vi "Inst_K2002.vi"(8 "error in":errorcluster, 10 "All Message Queues in":T1, 11 "Prueba31 in":refnum<class "Prueba31.lvclass">) -> (0 "error out":errorcluster)   [LabVIEW 2019, in "Prueba31.lvclass"]
uses:
  Prueba31.lvclass
  QMH/Message Queue/All Message Queues.ctl
  QMH/Message Queue/Message Cluster.ctl
  Prueba31.lvclass/Prueba31.ctl
  <vilib>/Utility/error.llb/Error Cluster From Error Code.vi
  QMH/Message Queue/Enqueue Message (Single).vi
  <vilib>/ErrorRing/Error Ring.xnode
  QMH/Message Queue/Message Queue.lvlib
  Instrumento/Keithley2002/Keithley2002.lvclass
panel:
  out "All States":string[](array[string])
  out "Actual State":string
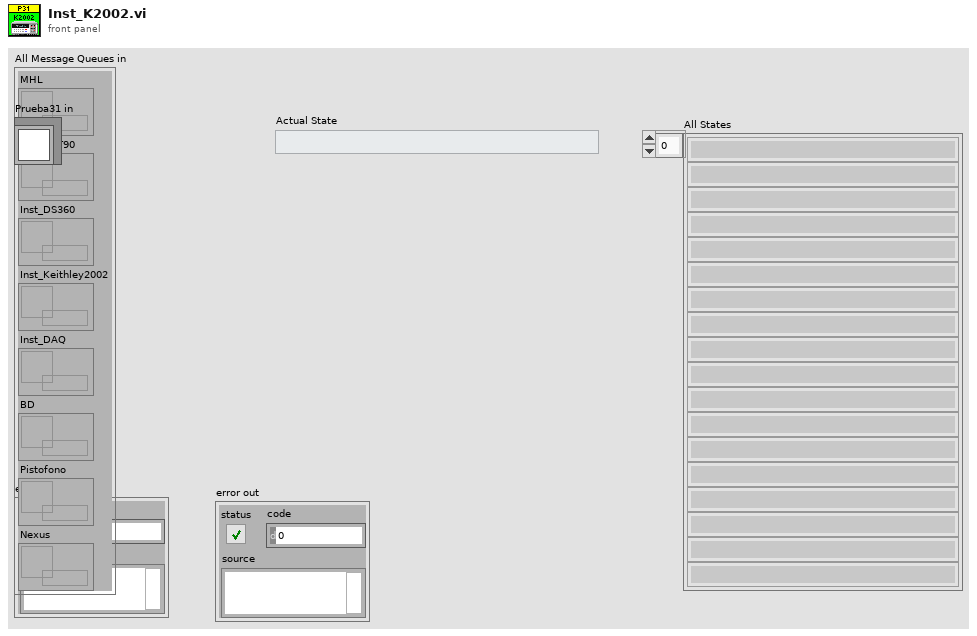
[diagram p1: front panel]
types:
  T1 = typedef "Message Queue.lvlib/All Message Queues.ctl" = cluster{"MHL":refnum<queue>, "Inst_CNT90":refnum<queue>, "Inst_DS360":refnum<queue>, "Inst_Keithley2002":refnum<queue>, "Inst_DAQ":refnum<queue>, "BD":refnum<queue>, "Pistofono":refnum<queue>, "Nexus":refnum<queue>}
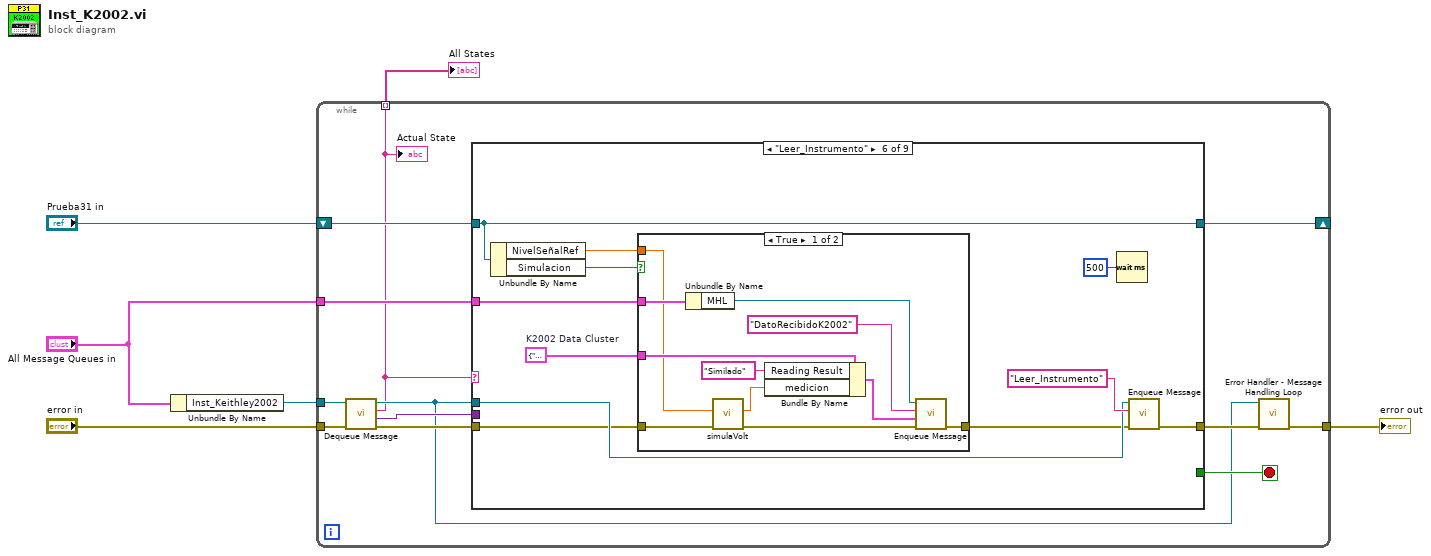
[diagram p0: block diagram]
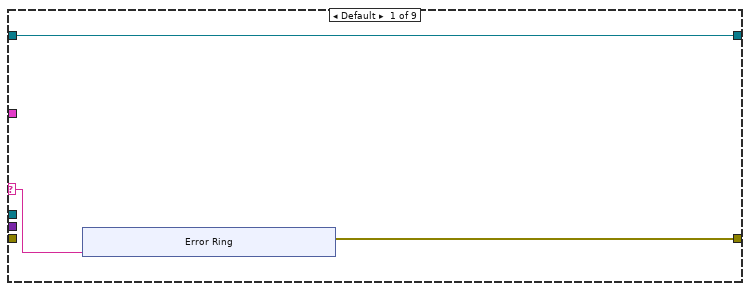
[diagram p2: hidden frame]
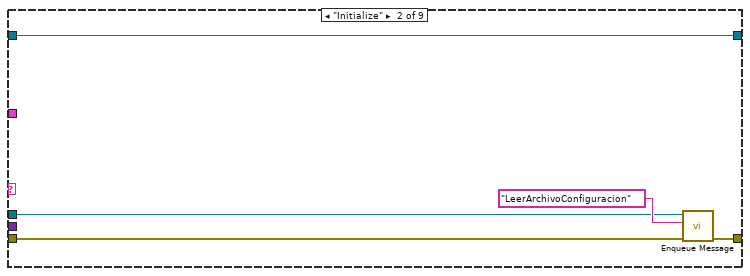
[diagram p3: hidden frame]
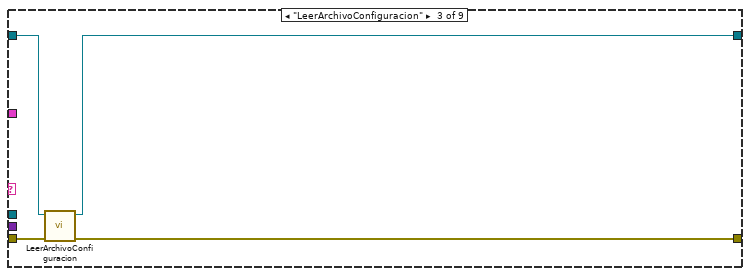
[diagram p4: hidden frame]
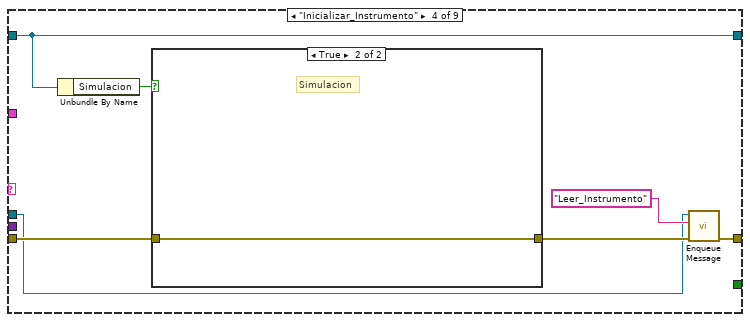
[diagram p5: hidden frame]
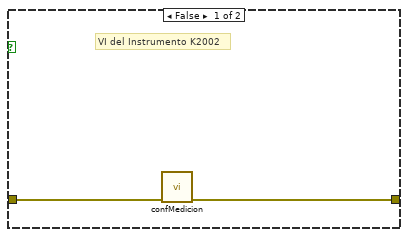
[diagram p6: hidden frame]
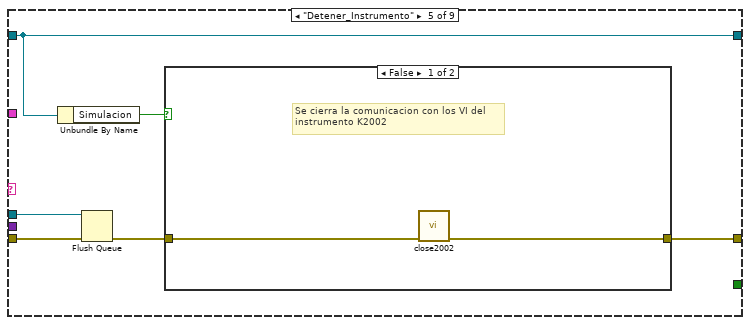
[diagram p7: hidden frame]
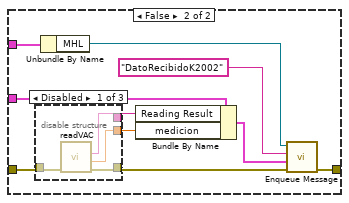
[diagram p9: hidden frame]
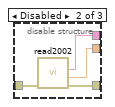
[diagram p10: hidden frame]
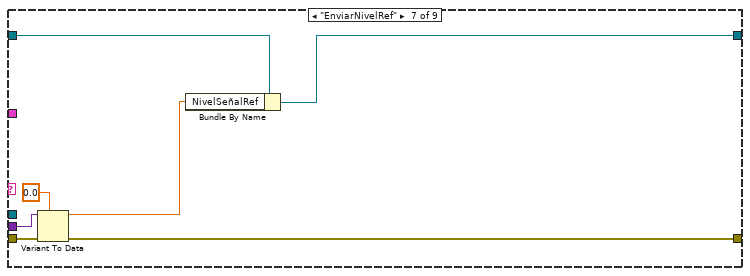
[diagram p12: hidden frame]
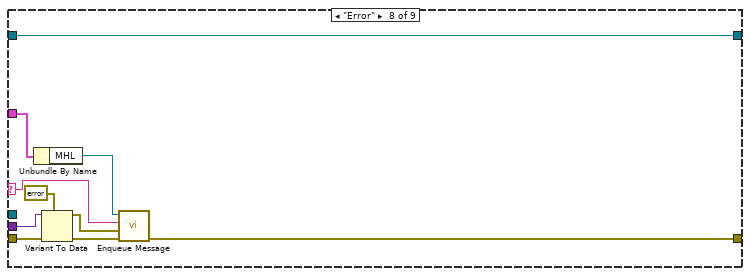
[diagram p13: hidden frame]
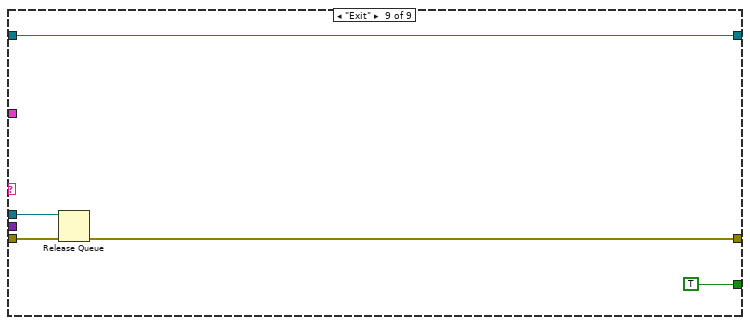
[diagram p14: hidden frame]
diagram:
  n1 = Unbundle By Name("All Message Queues in") -> ("Inst_Keithley2002"=w4:refnum<queue>)
  n2 = while {
    tunnel: "error in" -> [w18]
    tunnel: w4 -> [w17]
    tunnel: "All Message Queues in" -> [w16]
    tunnel: [w9] -> w2
    shift-right: [w12] -> _
    shift-left: "Prueba31 in" -> [w15]
    tunnel: [w7] -> w1 mode=indexing
    stop <- w11 stop-if-true
    n3 = call "Dequeue Message.vi"("error in (no error)"=w18, "Message Queue"=w17) -> ("error out"=w13:errorcluster, "Message Data"=w14:variant, "Message"=w7:string, "dup Message Queue"=w8:refnum<queue>)  [unwired: 6 in]
    "Actual State" <- w7
    n4 = case shown="\"Leer_Instrumento\"" w7 {
      selector: w7 -> [w21 _ _ _ _ _ _ w107 _]
      tunnel: w16 -> [_ _ _ _ _ w61 _ w106 _]
      tunnel: w15 -> [w19 w33 w34 w38 w52 w63 w99 w114 w116]
      tunnel: w8 -> [_ w29 _ w39 w50 w64 _ _ w118]
      tunnel: w14 -> [_ _ _ _ _ _ w101 w111 _]
      tunnel: w13 -> [_ w31 w36 w40 w48 w60 w103 w112 w119]
      tunnel: [w20 w30 w37 w41 w53 w65 w104 w109 w115] -> w10
      tunnel: [w19 w33 w35 w38 w52 w63 w100 w114 w116] -> w12
      tunnel: [_ _ _ _ _ _ _ _ TRUE] -> w11
      frame Default {
        n5 = xnode "Error Ring"("parameter 0"=w21) -> ("error out"=w20:errorcluster)
      }
      frame "Initialize" {
        n6 = call-poly "Enqueue Message.vi"("error in (no error)"=w31, "Message"="LeerArchivoConfiguracion", "Message Queue"=w29) -> ("error out"=w30:errorcluster)  [unwired: 7 in, 1 out]
      }
      frame "LeerArchivoConfiguracion" {
        n7 = call "LeerArchivoConfiguracion.vi"("error in"=w36, "Prueba31 in"=w34) -> ("error out"=w37:errorcluster, "Prueba31 out"=w35:refnum<class "Prueba31.lvclass">)  [unwired: 8 in]
      }
      frame "Inicializar_Instrumento" {
        n8 = Unbundle By Name(w38) -> ("Simulacion"=w43:bool)
        n9 = case shown="True" w43 {
          tunnel: [w46 w47] -> w44
          tunnel: w40 -> [w45 w47]
          frame False {
            # "VI del Instrumento K2002"
            n10 = call "confMedicion.vi"("error in (no error)"=w45) -> ("error out"=w46:errorcluster)  [unwired: 9 in, 1 out]
          }
          frame True {
            # "Simulacion"
          }
        }
        n11 = call-poly "Enqueue Message.vi"("error in (no error)"=w44, "Message"="Leer_Instrumento", "Message Queue"=w39) -> ("error out"=w41:errorcluster)  [unwired: 7 in, 1 out]
      }
      frame "Detener_Instrumento" {
        n12 = Unbundle By Name(w52) -> ("Simulacion"=w51:bool)
        n13 = Flush Queue(queue=w50, error in (no error)=w48) -> (error out=w49:errorcluster)  [unwired: 2 out]
        n14 = case shown="False" w51 {
          tunnel: [w55 w56] -> w53
          tunnel: w49 -> [w54 w56]
          frame False {
            # "Se cierra la comunicacion con los VI del\ninstrumento K2002"
            n15 = call "close2002.vi"("error in (no error)"=w54) -> ("error out"=w55:errorcluster)  [unwired: 9 in, 1 out]
          }
          frame True {
            # "Simulacion"
          }
        }
      }
      frame "Leer_Instrumento" {
        w58 = cluster{"Reading Result":string, "medicion":dbl} {"Reading Result"="", "medicion"=0.0}  # K2002 Data Cluster
        n16 = Unbundle By Name(w63) -> ("NivelSeñalRef"=w57:dbl, "Simulacion"=w62:bool)
        n17 = case shown="True" w62 {
          tunnel: w61 -> [w78 w88]
          tunnel: [w75 w87] -> w59
          tunnel: w60 -> [w77 w82]
          tunnel: w58 -> [w72 w84]
          tunnel: w57 -> [w68 _]
          frame True {
            n18 = Unbundle By Name(w78) -> ("MHL"=w74:refnum<queue>)
            n19 = call "simulaVolt.vi"("error in (no error)"=w77, "volt in"=w68) -> ("error out"=w76:errorcluster, "volt out"=w71:dbl)  [unwired: 7 in, 1 out]
            n20 = Bundle By Name(cluster=w72, "Reading Result"="Similado", "medicion"=w71) -> (w69:cluster{"Reading Result":string, "medicion":dbl})
            n21 = call-poly "Enqueue Message.vi"("error in (no error)"=w76, "Message Data"=w69, "Message"="DatoRecibidoK2002", "Message Queue"=w74) -> ("error out"=w75:errorcluster)  [unwired: 6 in, 1 out]
          }
          frame False {
            n22 = disable-structure shown="Disabled" {
              disable-tunnel: w82 -> [w92 w96 w97]
              disable-tunnel: [w91 w95 w97] -> w81
              disable-tunnel: [w90 w94 _] -> w80
              disable-tunnel: [w89 w93 _] -> w79
              frame Disabled {
                n23 = call "readVAC.vi"("error in (no error)"=w92) -> ("error out"=w91:errorcluster, "medicion"=w89:dbl, "Reading Result"=w90:string)  [unwired: 7 in, 1 out]
              }
              frame Disabled {
                n24 = call "read2002.vi"("error in (no error)"=w96) -> ("error out"=w95:errorcluster, "medicion"=w93:dbl, "Reading Result"=w94:string)  [unwired: 7 in, 1 out]
              }
              frame Enabled {
              }
            }
            n25 = Unbundle By Name(w88) -> ("MHL"=w86:refnum<queue>)
            n26 = Bundle By Name(cluster=w84, "Reading Result"=w80, "medicion"=w79) -> (w83:cluster{"Reading Result":string, "medicion":dbl})
            n27 = call-poly "Enqueue Message.vi"("error in (no error)"=w81, "Message Data"=w83, "Message"="DatoRecibidoK2002", "Message Queue"=w86) -> ("error out"=w87:errorcluster)  [unwired: 6 in, 1 out]
          }
        }
        n28 = Wait (ms)(milliseconds to wait=u32 500) -> ()  [unwired: 1 out]
        n29 = call-poly "Enqueue Message.vi"("error in (no error)"=w59, "Message"="Leer_Instrumento", "Message Queue"=w64) -> ("error out"=w65:errorcluster)  [unwired: 7 in, 1 out]
      }
      frame "EnviarNivelRef" {
        n30 = Variant To Data(error in=w103, type=0.0, Variant=w101) -> (data=w98:dbl, error out=w104:errorcluster)
        n31 = Bundle By Name(cluster=w99, "NivelSeñalRef"=w98) -> (w100:refnum<class "Prueba31.lvclass">)
      }
      frame "Error" {
        n32 = Unbundle By Name(w106) -> ("MHL"=w105:refnum<queue>)
        n33 = Variant To Data(error in=w112, type=errorcluster {"status"=FALSE, "code"=0, "source"=""} ("error constant"), Variant=w111) -> (data=w108:errorcluster, error out=w110:errorcluster)
        n34 = call-poly "Enqueue Message.vi"("error in (no error)"=w110, "Message Data"=w108, "Message"=w107, "Message Queue"=w105) -> ("error out"=w109:errorcluster)  [unwired: 6 in, 1 out]
      }
      frame "Exit" {
        n35 = Release Queue(queue=w118, error in (no error)=w119) -> (error out=w115:errorcluster)  [unwired: 1 in, 2 out]
      }
    }
    n36 = call "Error Handler - Message Handling Loop.vi"("error in (no error)"=w10, "Message Queue"=w8) -> ("dup error in"=w9:errorcluster)  [unwired: 8 in, 1 out]
  }
  "error out" <- w2
  "All States" <- w1
